vi "rad_MakeBackupFolder.vi"(3 "error in":errorcluster, 5 "ImagePathFolder":path) -> (0 "error out":errorcluster, 2 "BackupFolderPath":path)   [LabVIEW 2014]
panel:
  in  "backupFolderName":string="_backups"
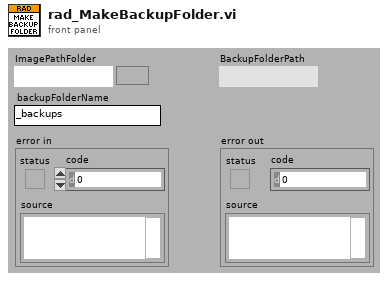
[diagram p1: front panel]
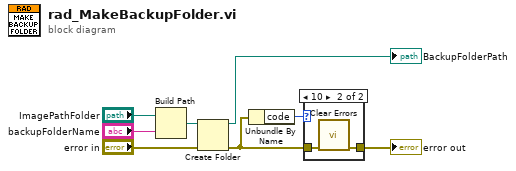
[diagram p0: block diagram]
diagram:
  n1 = Build Path(base path="ImagePathFolder", name or relative path="backupFolderName") -> (appended path=w2:path)
  n2 = Create Folder(path (use dialog)=w2, error in="error in") -> (created path=→"BackupFolderPath":path, error out=w6:errorcluster)  [unwired: 1 in, 1 out]
  n3 = Unbundle By Name(w6) -> ("code"=w5:i32)
  n4 = case shown="10" w5 {
    tunnel: [w9 w11] -> w7
    tunnel: w6 -> [w9 w10]
    frame 0, Default {
    }
    frame 10 {
      n5 = call <vilib>:"Clear Errors.vi"("error in (no error)"=w10) -> ("error out"=w11:errorcluster)  [unwired: 5 in, 1 out]
    }
  }
  "error out" <- w7
